vi "Set Error.vi"(8 "error in (no error)":errorcluster, 10 "errors":T1[](array[typedef]), 11 "DOM document in":refnum<k20>) -> (0 "error out":errorcluster, 3 "DOM document out":refnum<k20>)   [LabVIEW 2017, in "Error File Management.lvlib"]
uses:
  Error File Management.lvlib
  Controls/NI Error.ctl
  <vilib>/xml/Close Reference(Node).vi
  <vilib>/xml/NI_XML.lvlib
  <resource>/objmgr/DOMUserDefRef.rc
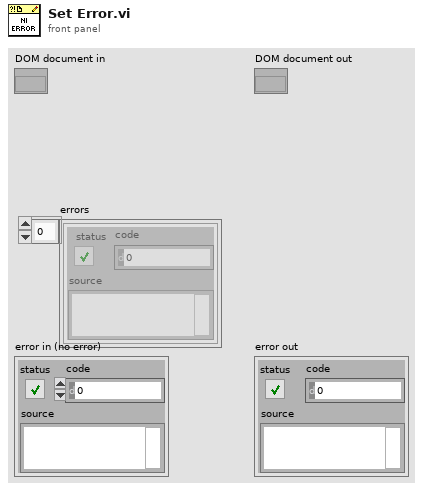
[diagram p1: front panel]
types:
  T1 = typedef "Error File Management.lvlib/NI Error.ctl" = errorcluster
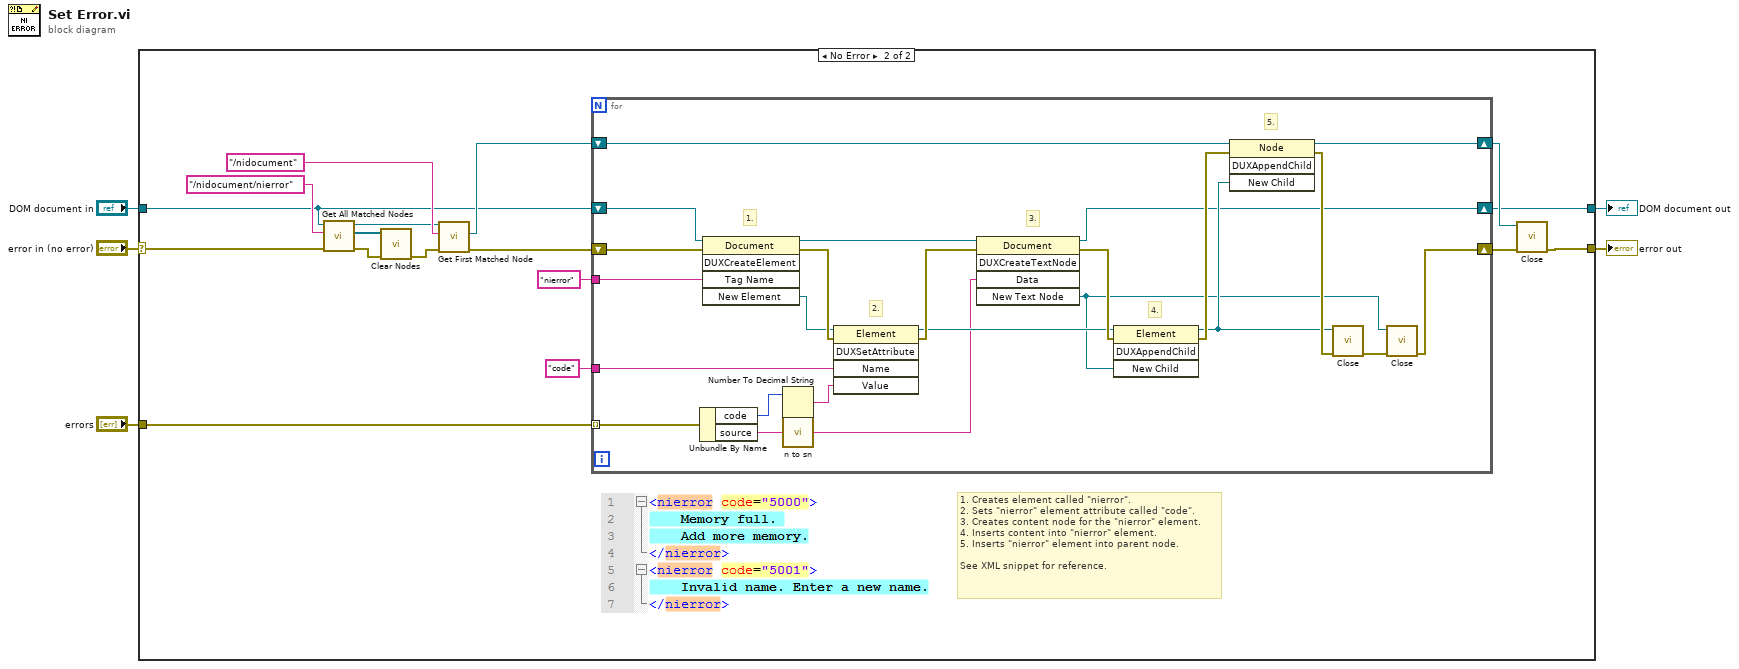
[diagram p0: block diagram]
diagram:
  n1 = case shown="No Error" "error in (no error)" {
    selector: "error in (no error)" -> [w7 w9]
    tunnel: "DOM document in" -> [w6 w12]
    tunnel: [w6 w11] -> w4
    tunnel: [w7 w10] -> w2
    tunnel: "errors" -> [_ w8]
    frame Error {
    }
    frame No Error {
      # "1. Creates element called \"nierror\".\n2. Sets \"nierror\" element attribute called \"code\".\n3. Creates content node for the \"nierror\" element.\n4. Inserts content into \"nierror\" element.\n5. Inserts \"nierror\" element into parent node.\n\nSee XML snippet for reference."
      n2 = call <vilib>:"Get All Matched Nodes.vi"("error in (no error)"=w9, "XPath expression"="/nidocument/nierror", "node in"=w12) -> ("error out"=w24:errorcluster, "node result array"=w23:refnum<k20>[], "node out"=w14:refnum<k20>)  [unwired: 6 in]
      n3 = call "Clear Nodes.vi"("error in (no error)"=w24, "nodes"=w23) -> ("error out"=w13:errorcluster)  [unwired: 9 in]
      n4 = call <vilib>:"Get First Matched Node.vi"("error in (no error)"=w13, "XPath expression"="/nidocument", "node in"=w14) -> ("error out"=w15:errorcluster, "node result"=w16:refnum<k20>)  [unwired: 6 in, 1 out]
      n5 = for {
        tunnel: w8 -> [w39] mode=indexing
        tunnel: "nierror" -> [w43]
        tunnel: "code" -> [w40]
        shift-right: [w26] -> w18
        shift-left: w15 -> [w42]
        shift-right: [w34] -> w19
        shift-left: w16 -> [w44]
        shift-right: [w28] -> w11
        shift-left: w12 -> [w29]
        # "5."
        # "4."
        # "3."
        # "2."
        # "1."
        n6 = Unbundle By Name(w39) -> ("code"=w38:i32, "source"=w36:string)
        n7 = invoke class="Document" method="DUXCreateElement"(reference=w29, error in=w42, "Tag Name"=w43) -> (reference out=w32:refnum<k20>, error out=w45:errorcluster, "New Element"=w41:refnum<k20>)  [unwired: 2 in, 2 out]
        n8 = Number To Decimal String(number=w38) -> (decimal integer string=w37:string)  [unwired: 1 in]
        n9 = call "n to sn.vi"("in"=w36) -> ("out"=w31:string)
        n10 = invoke class="Element" method="DUXSetAttribute"(reference=w41, error in=w45, "Name"=w40, "Value"=w37) -> (reference out=w33:refnum<k20>, error out=w47:errorcluster)  [unwired: 1 in, 3 out]
        n11 = invoke class="Document" method="DUXCreateTextNode"(reference=w32, error in=w47, "Data"=w31) -> (reference out=w28:refnum<k20>, error out=w46:errorcluster, "New Text Node"=w25:refnum<k20>)  [unwired: 2 in, 2 out]
        n12 = invoke class="Element" method="DUXAppendChild"(reference=w33, error in=w46, "New Child"=w25) -> (reference out=w30:refnum<k20>, error out=w48:errorcluster)  [unwired: 1 in, 2 out]
        n13 = invoke class="Node" method="DUXAppendChild"(reference=w44, error in=w48, "New Child"=w30) -> (reference out=w34:refnum<k20>, error out=w35:errorcluster)  [unwired: 1 in, 2 out]
        n14 = call-poly <vilib>:"Close.vi"("error in (no error)"=w35, "node"=w30) -> ("error out"=w27:errorcluster)  [unwired: 7 in]
        n15 = call-poly <vilib>:"Close.vi"("error in (no error)"=w27, "node"=w25) -> ("error out"=w26:errorcluster)  [unwired: 7 in]
      }
      n16 = call-poly <vilib>:"Close.vi"("error in (no error)"=w18, "node"=w19) -> ("error out"=w10:errorcluster)  [unwired: 7 in]
    }
  }
  "DOM document out" <- w4
  "error out" <- w2
